vi "QD_git_add.vi"(6 "Variant in":variant, 7 "Shift Pressed?":bool, 8 "error in (no error)":errorcluster, 10 "QD Combo Box Ref":refnum<vi>, 11 "QD Launch VI Ref":refnum<vi>) -> (0 "error out":errorcluster, 4 "Variant out":variant)   [LabVIEW 2020, in "AJ_QuickDrop_Git.lvlib"]
doc: "Write a 1-2 sentence description of the functionality of your plugin here. Replace the \"$\" below with the character you wish to assign as the default shortcut for this plugin. Do not add any text after the 'Default Shortcut' line below.\n\nDefault Shortcut - [$]"
uses:
  AJ_QuickDrop_Git.lvlib
panel:
  in  "Undo Name":string="Quick Drop Keyboard Shortcut"
  # "Do not change the connector pane of this VI.\n\nSee the block diagram for directions on how to use this template."
  # "Specify the name of the Undo transaction"
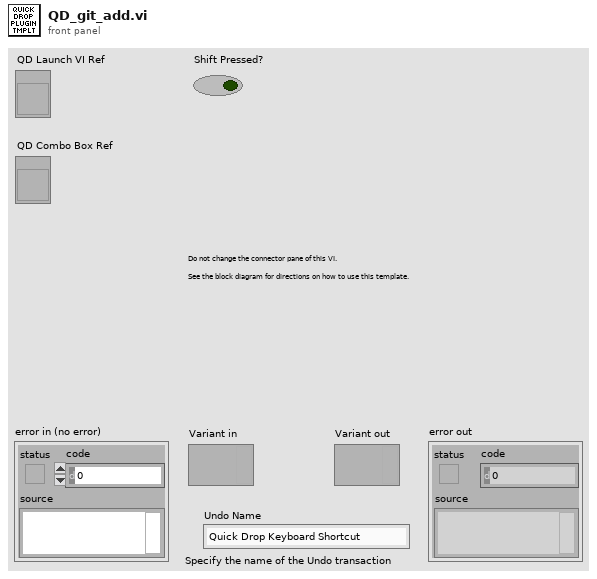
[diagram p1: front panel]
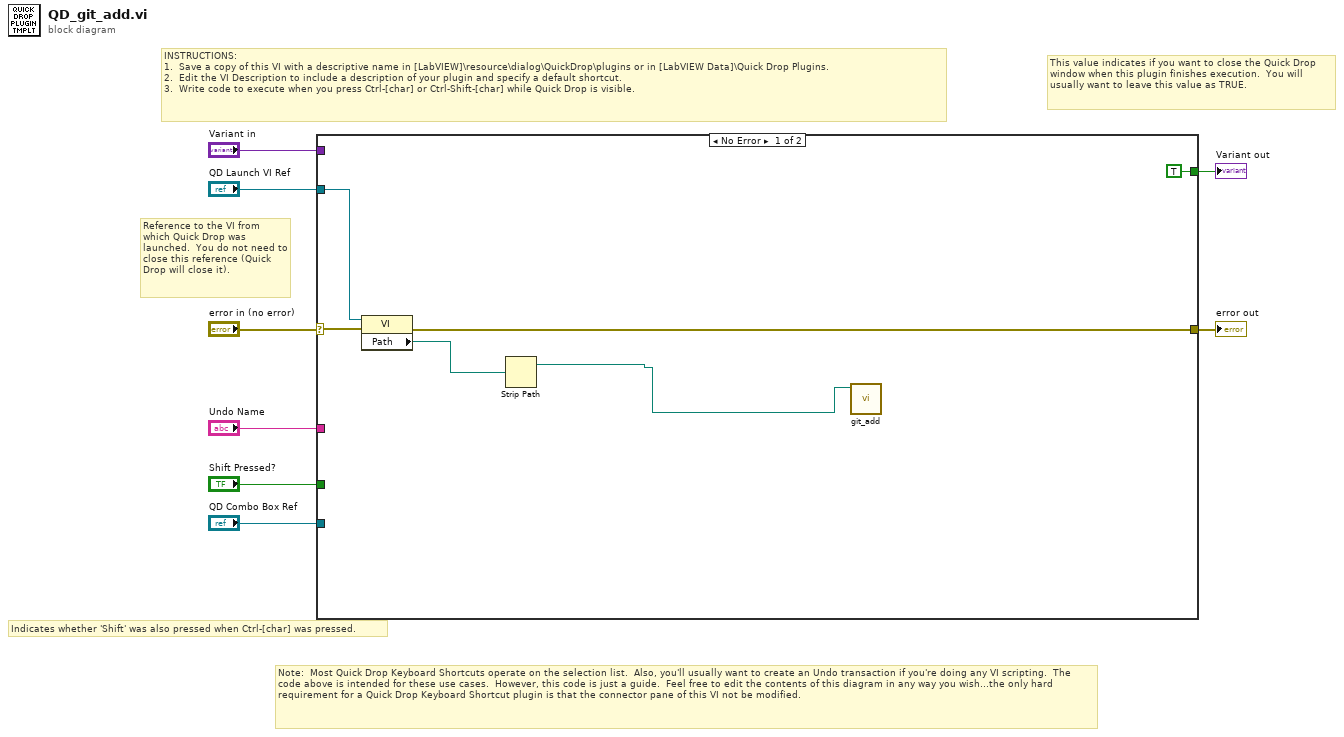
[diagram p0: block diagram]
diagram:
  # "Note:  Most Quick Drop Keyboard Shortcuts operate on the selection list.  Also, you'll usually want to create an Undo transaction if you're doing any VI scripting.  The code above is intended for these use cases.  However, this code is just a guide.  Feel free to edit the contents of this diagram in any way you wish...the only hard requirement for a Quick Drop Keyboard Shortcut plugin is that the connector pane of this VI not be modified."
  # "Indicates whether 'Shift' was also pressed when Ctrl-[char] was pressed."
  # "This value indicates if you want to close the Quick Drop window when this plugin finishes execution.  You will usually want to leave this value as TRUE."
  # "Reference to the VI from which Quick Drop was launched.  You do not need to close this reference (Quick Drop will close it)."
  # "INSTRUCTIONS:\n1.  Save a copy of this VI with a descriptive name in [LabVIEW]\\resource\\dialog\\QuickDrop\\plugins or in [LabVIEW Data]\\Quick Drop Plugins.\n2.  Edit the VI Description to include a description of your plugin and specify a default shortcut. \n3.  Write code to execute when you press Ctrl-[char] or Ctrl-Shift-[char] while Quick Drop is visible."
  n1 = case shown="No Error" "error in (no error)" {
    selector: "error in (no error)" -> [w14 w15]
    tunnel: [w11 w15] -> w7
    tunnel: "QD Launch VI Ref" -> [w13 _]
    tunnel: "Shift Pressed?" -> [_ _]
    tunnel: "QD Combo Box Ref" -> [_ _]
    tunnel: "Variant in" -> [_ _]
    tunnel: "Undo Name" -> [_ _]
    tunnel: [TRUE _] -> w1
    frame No Error {
      n2 = property class="VI"(reference=w13, error in=w14) -> (error out=w11:errorcluster, "Path"=w12:path)  [unwired: 1 out]
      n3 = Strip Path(path=w12) -> (stripped path=w9:path)  [unwired: 1 out]
      n4 = call <resource>:"git_add.vi"("Working Dir"=w9) -> ()  [unwired: 11 in]
    }
    frame Error {
    }
  }
  "error out" <- w7
  "Variant out" <- w1
